vi "VP.vi"(0 "OUTPUT VARS":refnum<vi>, 1 "INPUT VARS":refnum<vi>, 2 "States":refnum<vi>, 3 "VPStates":refnum<vi>, 4 "Processes":refnum<vi>, 5 "INP":refnum<vi>, 6 "PORTS":refnum<vi>) -> ()   [LabVIEW 2010]
uses:
  lib/Ports.lvclass
panel:
  in  "OUT Ports Array 2":cluster{"Порт":string, "Значение":bool[]}[](array[cluster])
  out "Здачения 2":string[](array[string])
  out "Типы 2":string[](array[string])
  out "Выходные глобальные переменные":string[](array[string])
  out "Значения":string[](array[string])
  out "Типы":string[](array[string])
  out "Входные глобальные переменные":string[](array[string])
  out "Cluster":T1
  in  "VPInputMsgs":refnum<vi>
  in  "SCM2VP":refnum<vi>
  out "Входные  сообщения для ВОУ":T2(array[cluster])
  in  "OUTP":refnum<vi>
  out "Состояния процессов":string[][](table)
  in  "OUT Ports Array":cluster{"Порт":string, "Значение":bool[]}[](array[cluster])
  # "Алгоритм управления"
  # "Значения входных портов"
  # "Значения выходных портов"
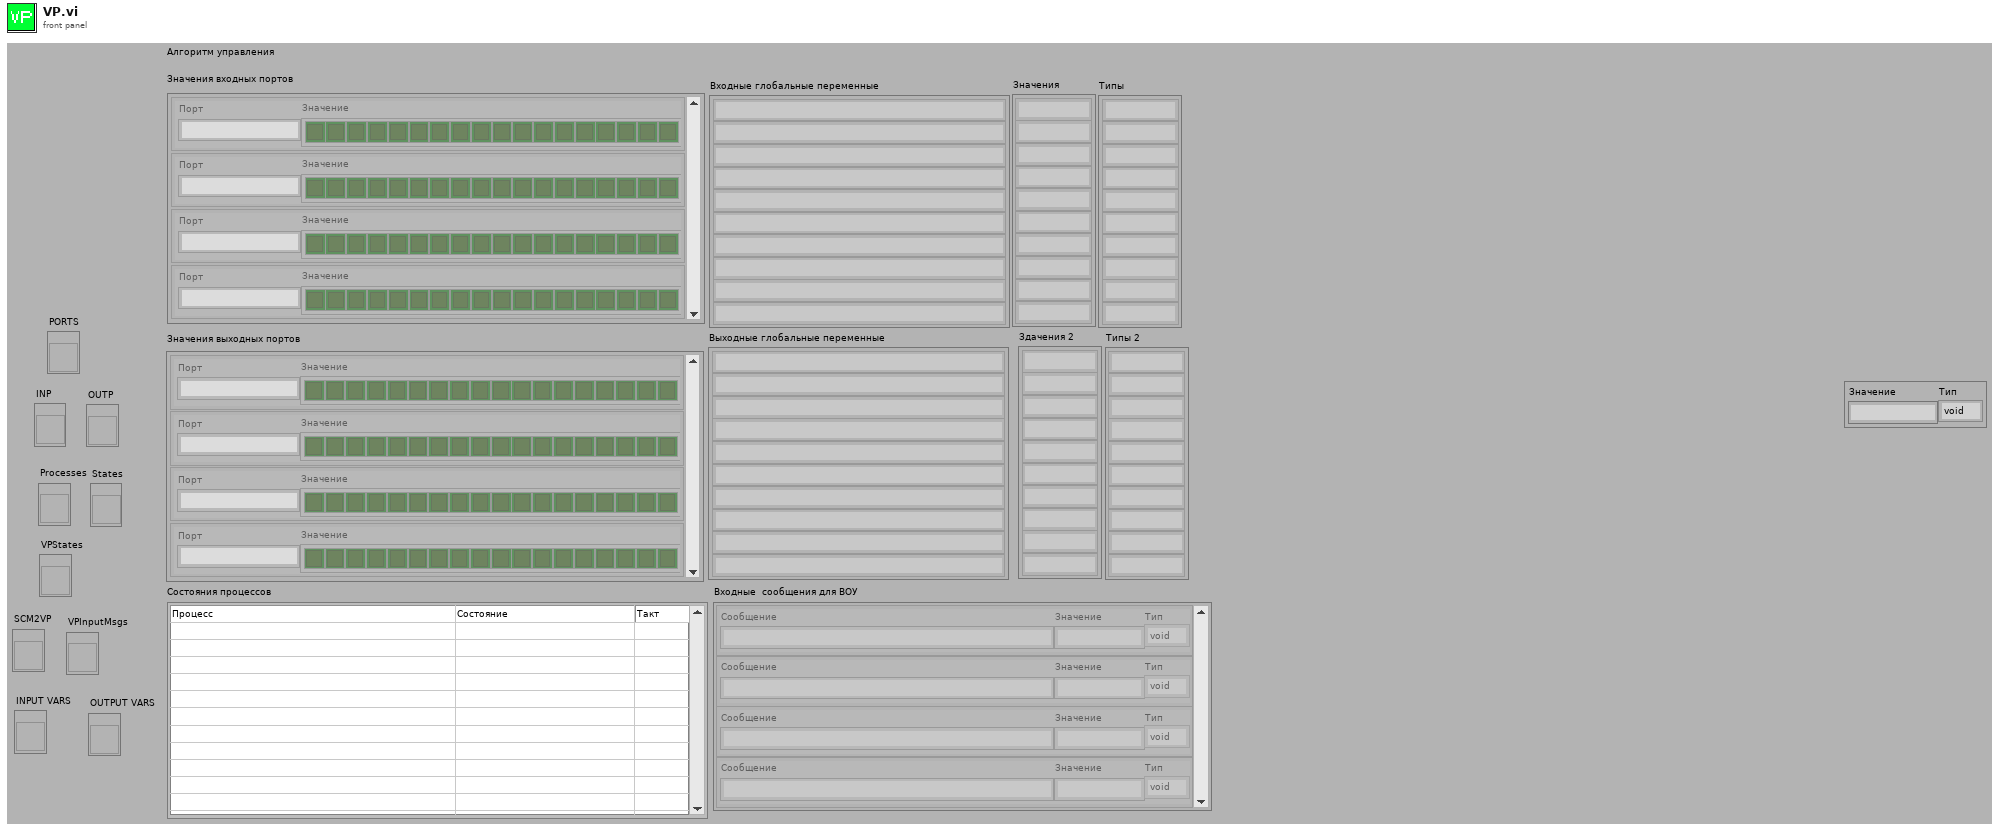
[diagram p1: front panel]
types:
  T1 = cluster{"Значение":string, "Тип":enum16{"void", "byte", "int", "float"}}
  T2 = cluster{"Сообщение":string, "Значение":string, "Тип":enum16{"void", "byte", "int", "float"}}[]
  T3 = cluster{"Сообщение":string, "Значение":string, "Тип":enum16{"void", "byte", "int", "float"}}
  T4 = cluster{"Input varables names":string[], "Input varables type":string[], "Input varables ports":i32[], "Input varables bytes":i32[]}
  T5 = cluster{"Output varables names":string[], "Output varables type":string[], "Output varables ports":i32[], "Output varables bytes":i32[]}
  T6 = cluster{"CA Output Numbers ":i32[], "CA Input Numbers":i32[], "VP Input Names":string[], "VP Output Names ":string[]}
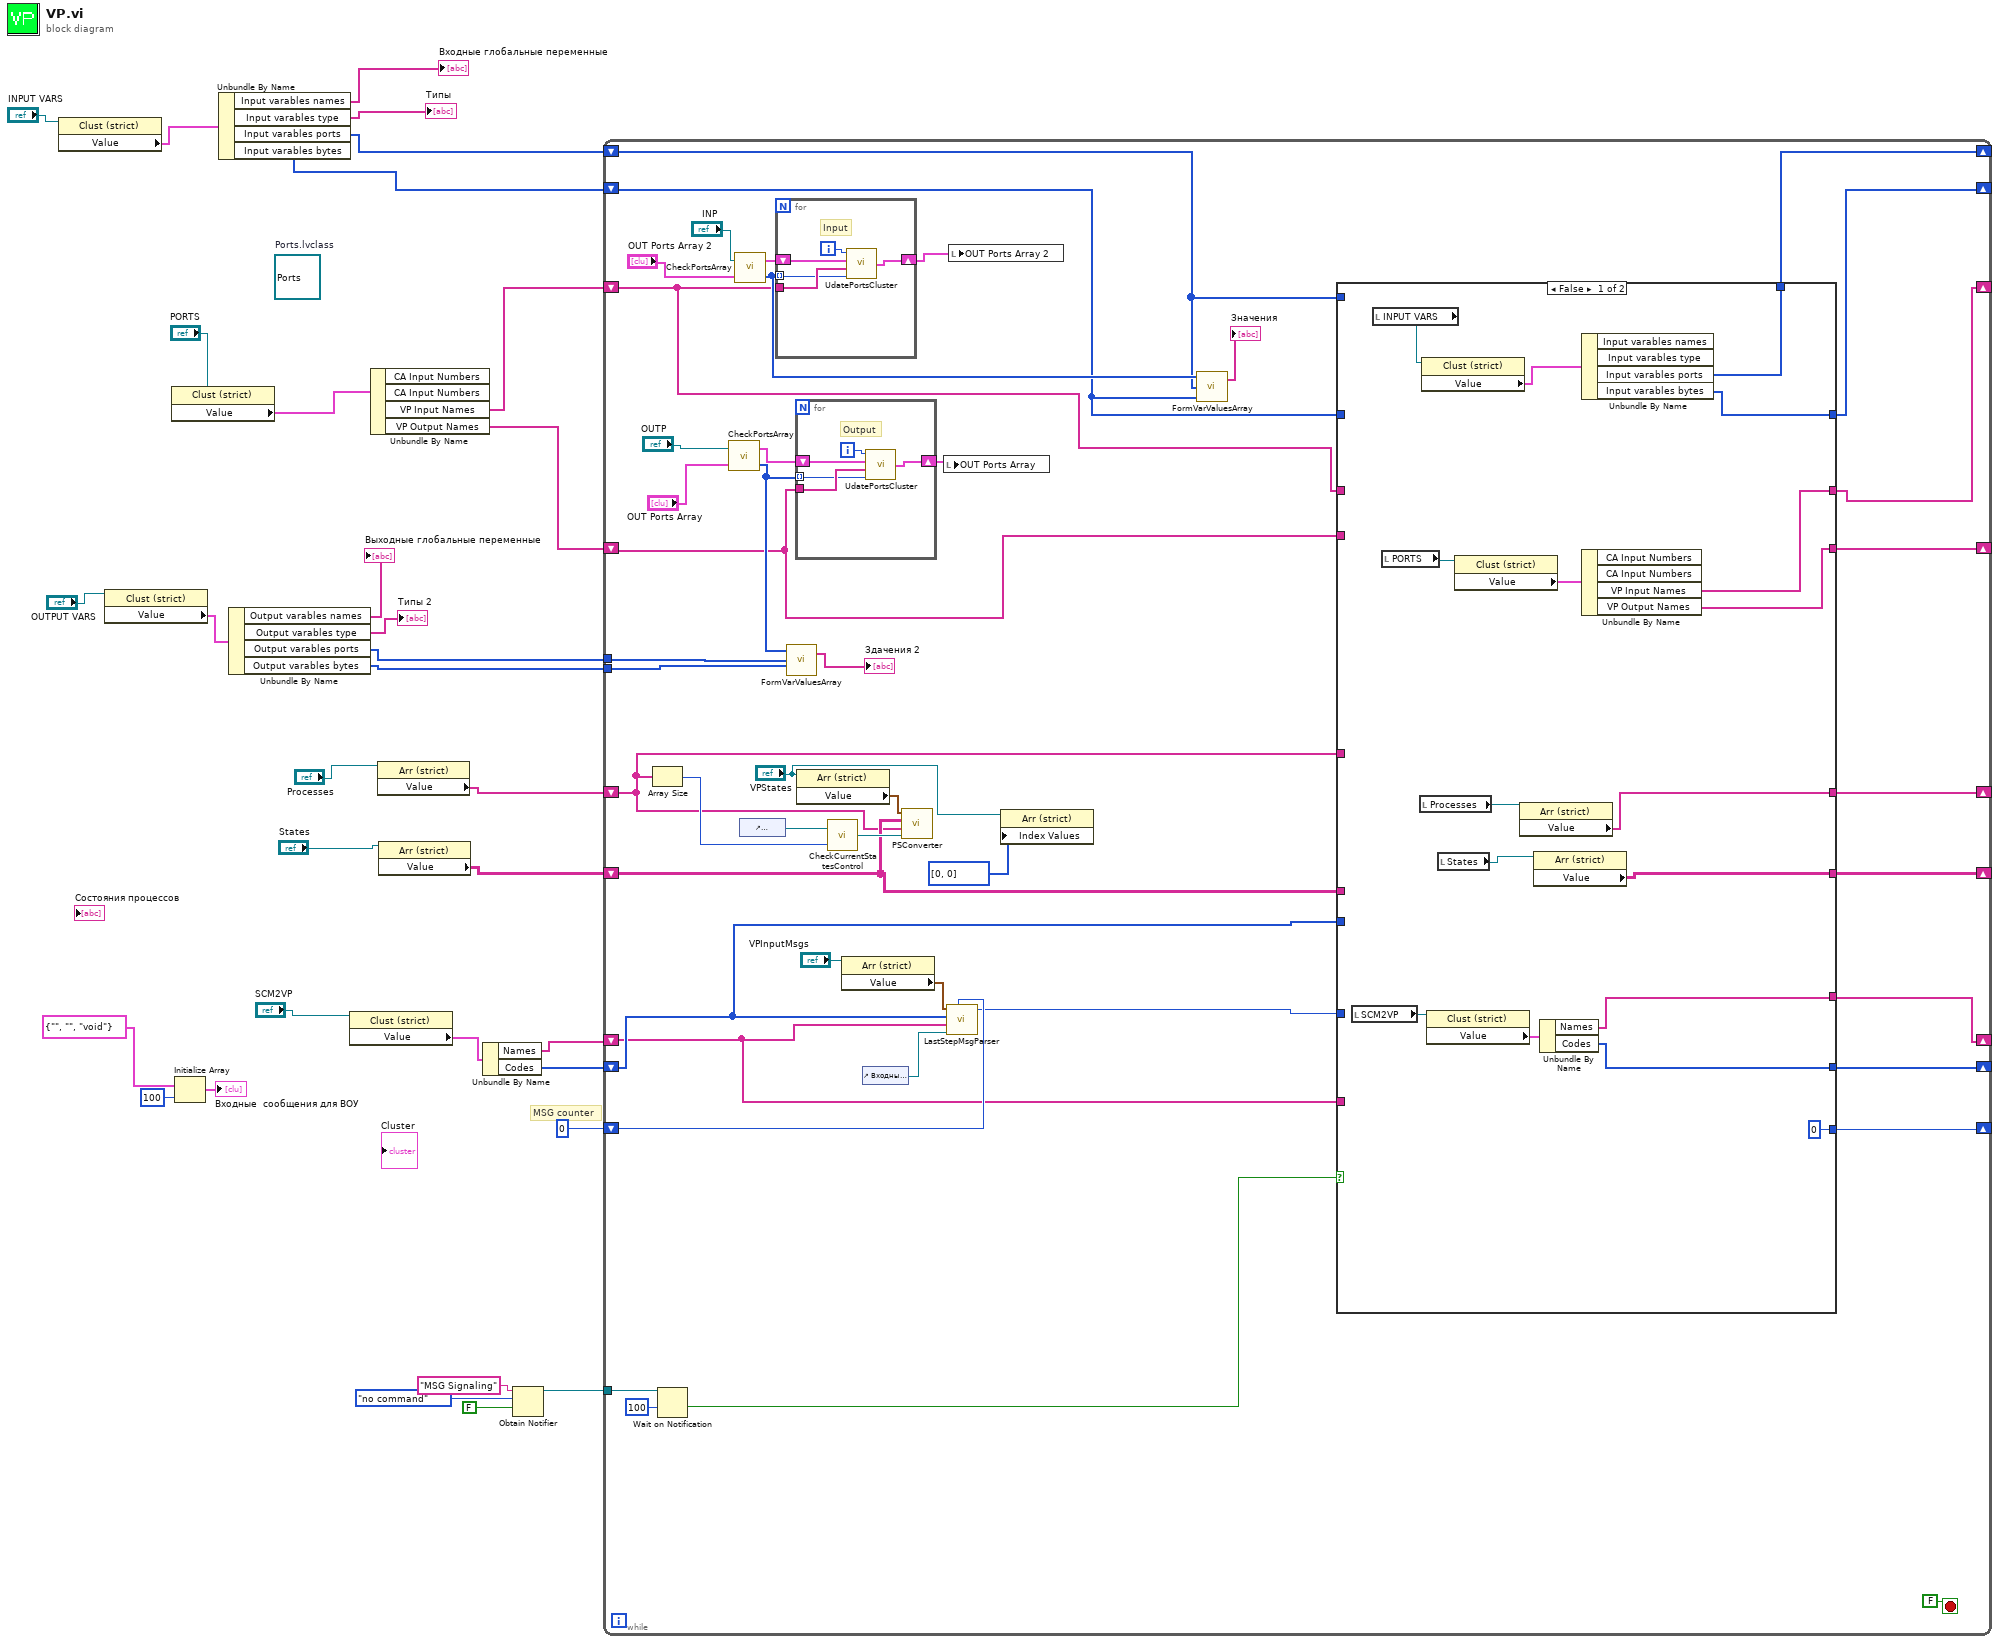
[diagram p0: block diagram]
diagram:
  (unwired) refnum<class "Ports.lvclass"> refnum  # Ports.lvclass
  # "MSG counter"
  n1 = property class="Clust (strict)"(reference="INPUT VARS") -> ("Value"=w16:T4)  [unwired: 1 in, 2 out]
  n2 = property class="Clust (strict)"(reference="OUTPUT VARS") -> ("Value"=w9:T5)  [unwired: 1 in, 2 out]
  n3 = property class="Clust (strict)"(reference="PORTS") -> ("Value"=w31:T6)  [unwired: 1 in, 2 out]
  n4 = Initialize Array(T3 {"Сообщение"="", "Значение"="", "Тип"=enum."void"} ("Cluster"), 100 ("dimension size")) -> (→"Входные  сообщения для ВОУ":T2)
  n5 = Unbundle By Name(w16) -> ("Input varables names"=→"Входные глобальные переменные":string[], "Input varables type"=→"Типы":string[], "Input varables ports"=w15:i32[], "Input varables bytes"=w14:i32[])
  n6 = Unbundle By Name(w9) -> ("Output varables names"=→"Выходные глобальные переменные":string[], "Output varables type"=→"Типы 2":string[], "Output varables ports"=w6:i32[], "Output varables bytes"=w5:i32[])
  n7 = property class="Clust (strict)"(reference="SCM2VP") -> ("Value"=w24:cluster{"Names":string[], "Codes":i32[]})  [unwired: 1 in, 2 out]
  n8 = Unbundle By Name(w31) -> ("VP Input Names"=w30:string[], "VP Output Names"=w11:string[])  [unwired: 2 out]
  n9 = property class="Arr (strict)"(reference="Processes") -> ("Value"=w27:string[])  [unwired: 1 in, 2 out]
  n10 = property class="Arr (strict)"(reference="States") -> ("Value"=w26:string[][])  [unwired: 1 in, 2 out]
  n11 = Unbundle By Name(w24) -> ("Names"=w23:string[], "Codes"=w22:i32[])
  n12 = Obtain Notifier(name (unnamed)="MSG Signaling", notification data type=enum16{"no command", "refresh"}."no command", create if not found? (T)=FALSE) -> (notifier out=w1:refnum<notifier>)  [unwired: 1 in, 2 out]
  n13 = while {
    shift-right: [w53] -> _
    shift-left: 0 ("dimension size") -> [w63]
    tunnel: w6 -> [w60]
    tunnel: w5 -> [w59]
    tunnel: w1 -> [w56]
    shift-right: [w51] -> _
    shift-left: w22 -> [w52]
    shift-right: [w50] -> _
    shift-left: w23 -> [w49]
    shift-right: [w44] -> _
    shift-left: w26 -> [w47]
    shift-right: [w45] -> _
    shift-left: w27 -> [w46]
    shift-right: [w36] -> _
    shift-left: w14 -> [w42]
    shift-right: [w37] -> _
    shift-left: w15 -> [w43]
    shift-right: [w39] -> _
    shift-left: w11 -> [w40]
    shift-right: [w38] -> _
    shift-left: w30 -> [w41]
    stop <- FALSE ("stop") stop-if-true
    n14 = Array Size(array=w46) -> (size(s)=w48:i32)
    n15 = Wait on Notification(notifier=w56, timeout in ms (-1)=100) -> (timed out?=w55:bool)  [unwired: 2 in, 3 out]
    n16 = call "CheckPortsArray.vi"("INP Ports Array 2"="OUT Ports Array", "INP"="OUTP") -> ("Value"=w58:i8[], "INP Ports Array"=w74:cluster{"String":string, "Array 2":bool[]}[])
    n17 = call "CheckPortsArray.vi"("INP Ports Array 2"="OUT Ports Array 2", "INP"="INP") -> ("Value"=w62:i8[], "INP Ports Array"=w77:cluster{"String":string, "Array 2":bool[]}[])
    n18 = control-ref of="Состояния процессов"() -> (w71:refnum<vi>)
    n19 = for {
      tunnel: w62 -> [w113] mode=indexing
      tunnel: w41 -> [w114]
      shift-right: [w110] -> w33
      shift-left: w77 -> [w111]
      i -> [w112]
      # "Input"
      n20 = call "UdatePortsCluster.vi"("Numeric 2"=w113, "Input Names"=w114, "Ports Array"=w111, "index"=w112) -> ("INP Ports Array 2"=w110:cluster{"String":string, "Array 2":bool[]}[])
    }
    n21 = call "FormVarValuesArray.vi"("varables bytes"=w59, "varables ports"=w60, "Ports"=w58) -> ("Values Array"=→"Здачения 2":string[])  [unwired: 1 in]
    n22 = for {
      tunnel: w58 -> [w108] mode=indexing
      tunnel: w40 -> [w109]
      shift-right: [w105] -> w73
      shift-left: w74 -> [w106]
      i -> [w107]
      # "Output"
      n23 = call "UdatePortsCluster.vi"("Numeric 2"=w108, "Input Names"=w109, "Ports Array"=w106, "index"=w107) -> ("INP Ports Array 2"=w105:cluster{"String":string, "Array 2":bool[]}[])
    }
    n24 = property class="Arr (strict)"(reference="VPStates") -> ("Value"=w72:cluster{"TimeInState":u16, "cur_state":i8}[])  [unwired: 1 in, 2 out]
    n25 = call "CheckCurrentStatesControl.vi"("Processes"=w48, "Inp reference"=w71) -> ("Out Refnum"=w70:refnum<vi>)
    n26 = property class="Arr (strict)"(reference="VPInputMsgs") -> ("Value"=w65:cluster{"MSG":i16, "param":i32, "Type":i16}[])  [unwired: 1 in, 2 out]
    n27 = control-ref of="Входные  сообщения для ВОУ"() -> (w64:refnum<vi>)
    n28 = call "PSConverter.vi"("Tbl Refnum"=w70, "PROC"=w46, "STATES"=w47, "Input claster"=w72) -> ()  [unwired: 1 out]
    n29 = local write "OUT Ports Array"(w73) -> ()
    n30 = call "LastStepMsgParser.vi"("Arr Refnum"=w64, "Out MSG Names"=w49, "old msg counter"=w63, "Codes"=w52, "Msg Array"=w65) -> ("current msg counter"=w54:i32)  [unwired: 4 in, 1 out]
    n31 = local write "OUT Ports Array 2"(w33) -> ()
    n32 = property class="Arr (strict)"(reference="VPStates", "Index Values"=u32[] [0, 0]) -> ()  [unwired: 1 in, 2 out]
    n33 = call "FormVarValuesArray.vi"("varables bytes"=w42, "varables ports"=w43, "Ports"=w62) -> ("Values Array"=→"Значения":string[])  [unwired: 1 in]
    n34 = case shown="False" w55 {
      tunnel: w54 -> [_ w102]
      tunnel: [0 ("current msg counter") w102] -> w53
      tunnel: w52 -> [_ w104]
      tunnel: [w91 w104] -> w51
      tunnel: [w92 w103] -> w50
      tunnel: w49 -> [_ w103]
      tunnel: w47 -> [_ w100]
      tunnel: w46 -> [_ w101]
      tunnel: [w89 w101] -> w45
      tunnel: [w87 w100] -> w44
      tunnel: w40 -> [_ w99]
      tunnel: w43 -> [_ w97]
      tunnel: w42 -> [_ w96]
      tunnel: w41 -> [_ w98]
      tunnel: [w84 w99] -> w39
      tunnel: [w83 w98] -> w38
      tunnel: [w80 w97] -> w37
      tunnel: [w79 w96] -> w36
      frame False {
        n35 = local read "SCM2VP"() -> (w94:refnum<vi>)
        n36 = local read "INPUT VARS"() -> (w81:refnum<vi>)
        n37 = local read "PORTS"() -> (w85:refnum<vi>)
        n38 = local read "Processes"() -> (w90:refnum<vi>)
        n39 = property class="Clust (strict)"(reference=w81) -> ("Value"=w82:T4)  [unwired: 1 in, 2 out]
        n40 = property class="Clust (strict)"(reference=w94) -> ("Value"=w93:cluster{"Names":string[], "Codes":i32[]})  [unwired: 1 in, 2 out]
        n41 = local read "States"() -> (w88:refnum<vi>)
        n42 = property class="Clust (strict)"(reference=w85) -> ("Value"=w86:T6)  [unwired: 1 in, 2 out]
        n43 = property class="Arr (strict)"(reference=w90) -> ("Value"=w89:string[])  [unwired: 1 in, 2 out]
        n44 = property class="Arr (strict)"(reference=w88) -> ("Value"=w87:string[][])  [unwired: 1 in, 2 out]
        n45 = Unbundle By Name(w93) -> ("Names"=w92:string[], "Codes"=w91:i32[])
        n46 = Unbundle By Name(w82) -> ("Input varables ports"=w80:i32[], "Input varables bytes"=w79:i32[])  [unwired: 2 out]
        n47 = Unbundle By Name(w86) -> ("VP Input Names"=w83:string[], "VP Output Names"=w84:string[])  [unwired: 2 out]
      }
      frame True {
      }
    }
  }
